vi "Com_Test.vi"() -> ()   [LabVIEW 2020]
uses:
  <vilib>/Instr/_visa.llb/VISA Configure Serial Port (Serial Instr).vi
panel:
  out "missed msg":u16
  out "error out":errorcluster
  out "error cleared?":bool
  out "Next Cmd":enum16{"getParm", "inc", "mph", "err"}(ring)
  out "Next State":enum16{"Initialize", "Send", "Receive", "Error"}(ring)
  out "stopping":bool
  out "Target MPH":u16 max=12 step=1 format="%2d"
  out "step":i32
  out "Target INC":u16 max=12 step=1
  out "Speed Changed":bool
  out "Inc Changed":bool
  in  "stop":bool
  out "read buffer":string
  out "refnum out":refnum<file>
  out "MPH READ":u8
  out "MPH READ 2":u8
  out "INC READ":u8
  out "INC READ 2":u8
  out "PD READ":u8 format="%x"
  out "PD READ 2":u8 format="%x"
  in  "Serial Port":refnum<visa-resource-name>="COM8"
  out "FootPath":path
  out "FootPathRef":refnum<file>
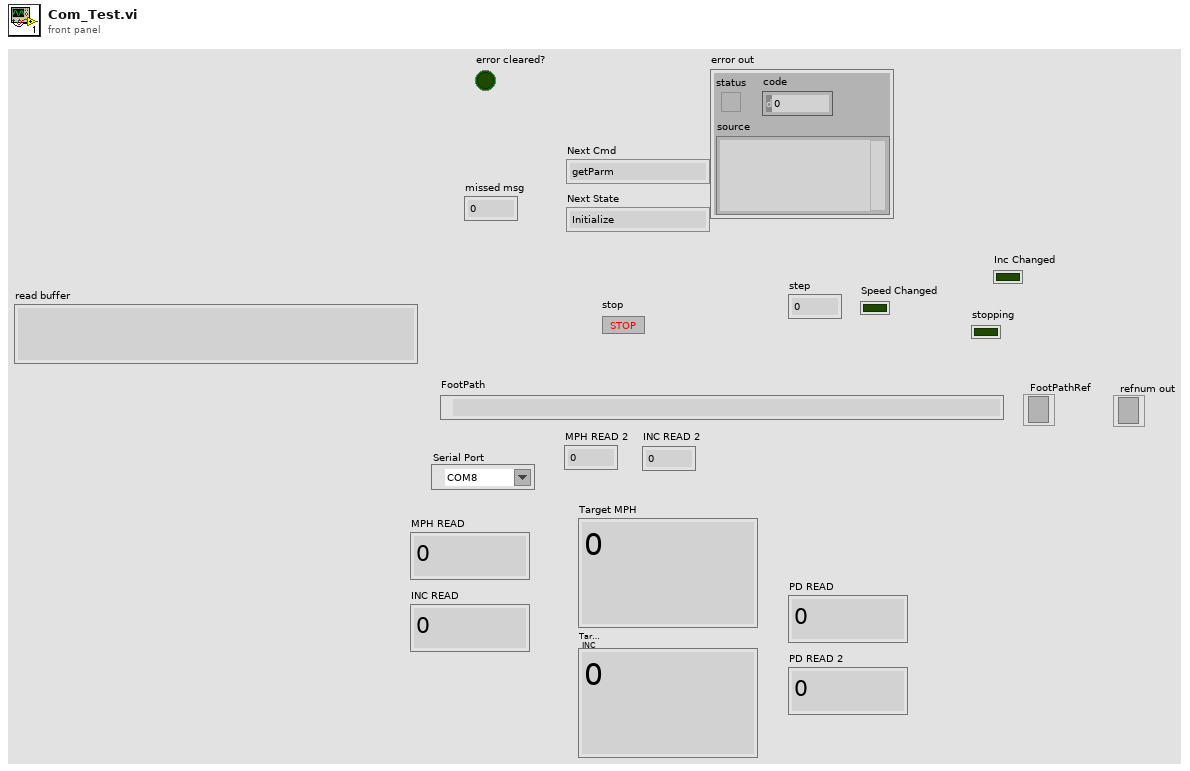
[diagram p1: front panel]
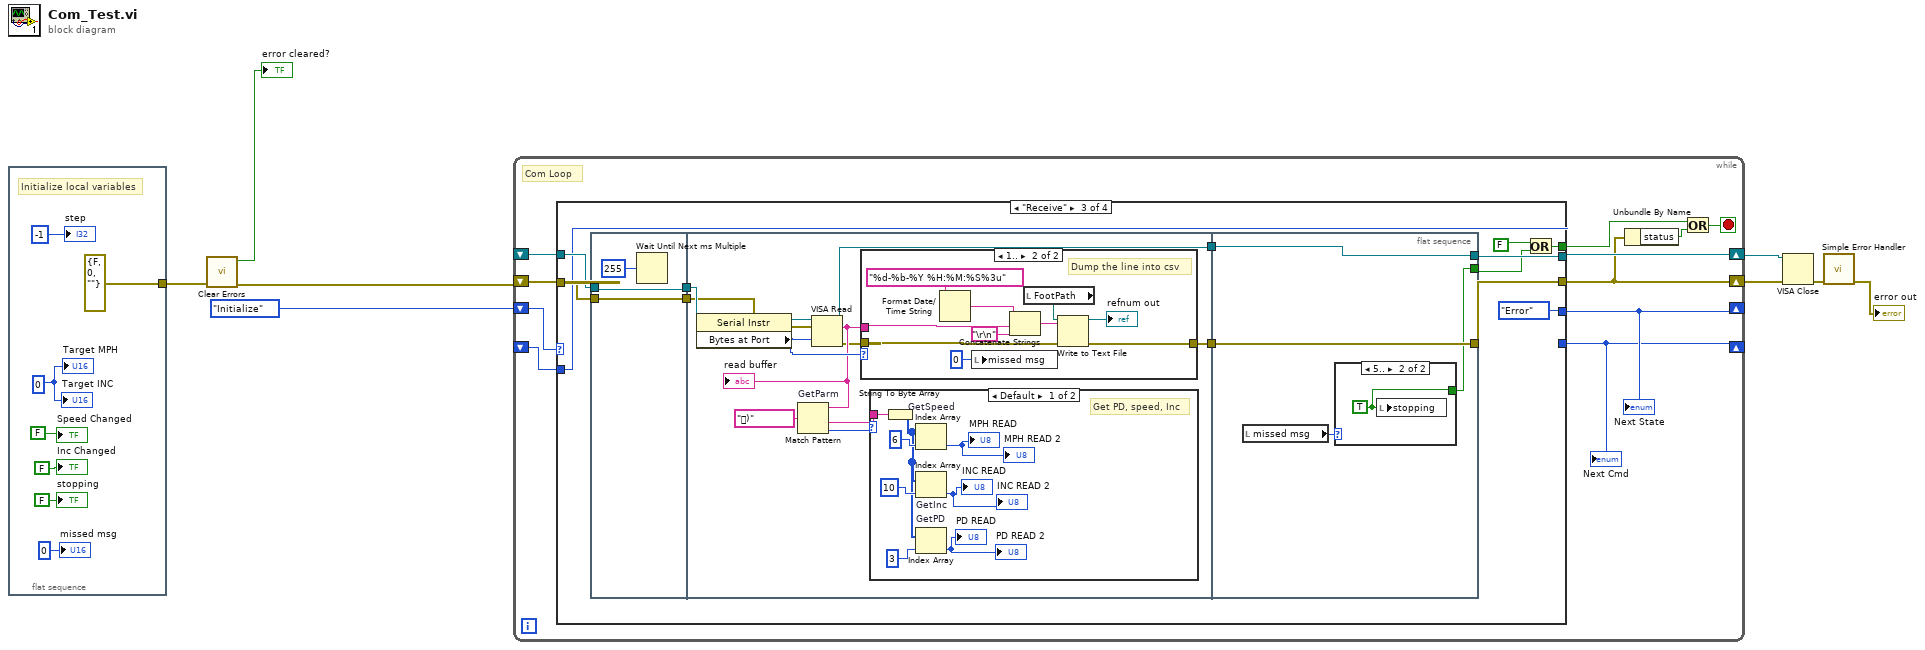
[diagram p0: block diagram]
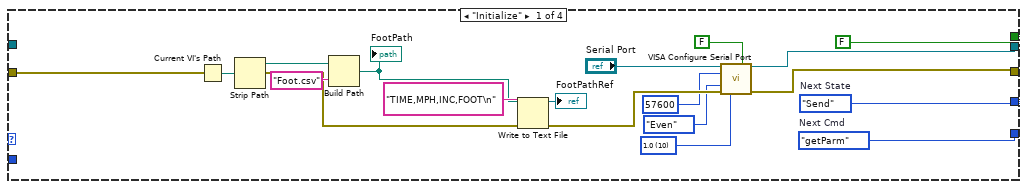
[diagram p2: hidden frame]
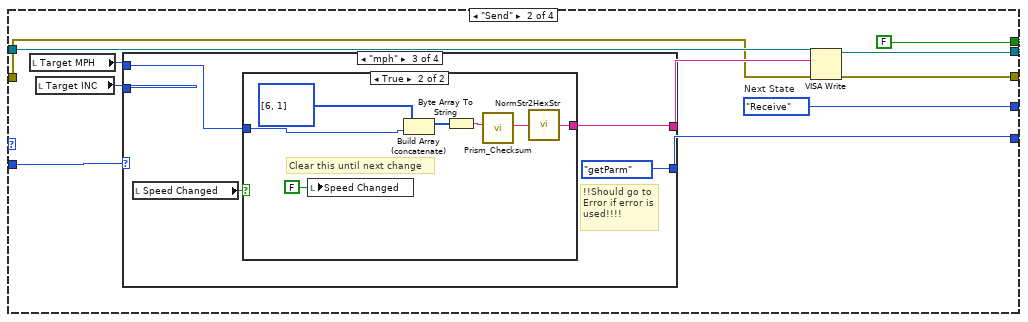
[diagram p3: hidden frame]
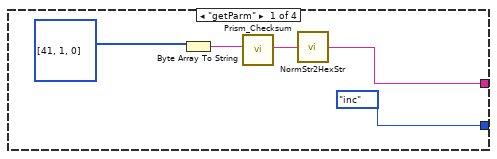
[diagram p4: hidden frame]
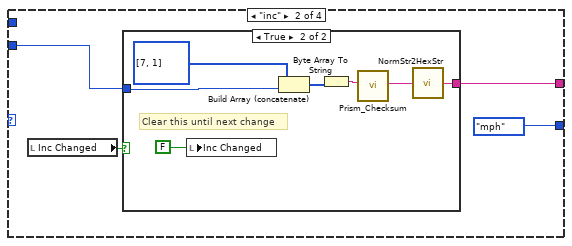
[diagram p5: hidden frame]
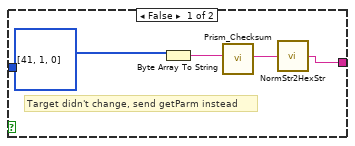
[diagram p6: hidden frame]
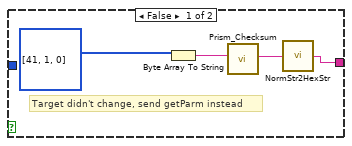
[diagram p7: hidden frame]
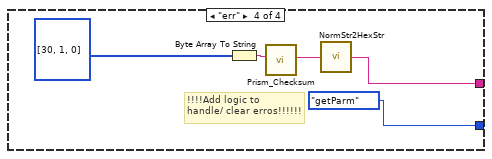
[diagram p8: hidden frame]
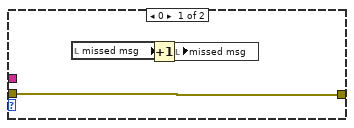
[diagram p10: hidden frame]
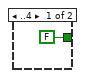
[diagram p11: hidden frame]
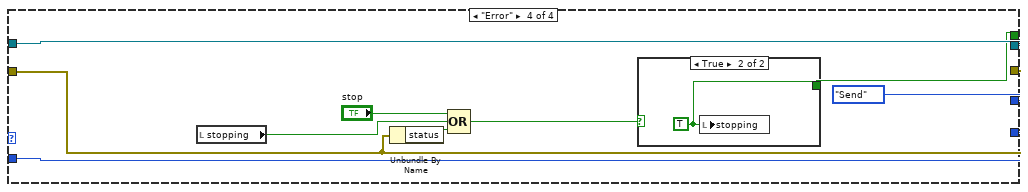
[diagram p12: hidden frame]
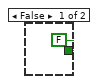
[diagram p13: hidden frame]
diagram:
  n1 = flat-sequence {
    tunnel: [errorcluster {"status"=FALSE, "code"=0, "source"=""} ("error constant")] -> w4
    frame #0 {
      w11 = u16 0 ("MPH")
      # "Initialize local variables"
      "stopping" <- FALSE ("stopping")
      "Target MPH" <- w11
      "step" <- -1 ("step")
      "Target INC" <- w11
      "Speed Changed" <- FALSE ("Value Changed")
      "Inc Changed" <- FALSE ("Inc Changed")
      "missed msg" <- u16 0 ("0 bytes")
    }
  }
  n2 = call <vilib>:"Clear Errors.vi"("error in (no error)"=w4) -> ("error out"=w3:errorcluster, "specific error cleared?"=→"error cleared?":bool)  [unwired: 5 in]
  n3 = while {
    shift-right: [w18] -> w7
    shift-left: w3 -> [w26]
    shift-right: [w23] -> w6
    shift-left: _ -> [w25]
    shift-right: [w22] -> _
    shift-left: enum16{"Initialize", "Send", "Receive", "Error"}."Initialize" ("Next State") -> [w24]
    shift-right: [w21] -> _
    shift-left: _ -> [w20]
    stop <- w17 stop-if-true
    # "Com Loop"
    n4 = case shown="\"Receive\"" w24 {
      tunnel: w26 -> [w32 w46 w106 w152]
      tunnel: w25 -> [_ w53 w108 w157]
      tunnel: [w42 w55 w101 w157] -> w23
      tunnel: [w41 w54 w102 w152] -> w18
      tunnel: [w38 w49 enum16{"Initialize", "Send", "Receive", "Error"}."Error" enum16{"Initialize", "Send", "Receive", "Error"}."Send"] -> w22
      tunnel: [w40 w47 w105 w158] -> w21
      tunnel: w20 -> [_ w45 w105 w158]
      tunnel: [FALSE FALSE w98 w153] -> w19
      frame "Initialize" {
        w27 = u16 10 items=["1.0"=10, "1.5"=15, "2.0"=20] ("stop bits (10: 1 bit)")
        w38 = enum16{"Initialize", "Send", "Receive", "Error"}."Send"  # Next State
        w40 = enum16{"getParm", "inc", "mph", "err"}."getParm"  # Next Cmd
        n5 = Current VI's Path() -> (path=w37:path)
        n6 = Strip Path(path=w37) -> (stripped path=w36:path)  [unwired: 1 out]
        n7 = Build Path(base path=w36, name or relative path="Foot.csv") -> (appended path=w33:path)
        "FootPath" <- w33
        n8 = Write to Text File(file (use dialog)=w33, text="TIME,MPH,INC,FOOT\n", error in=w32) -> (refnum out=→"FootPathRef":refnum<file>, error out=w31:errorcluster)  [unwired: 1 in, 1 out]
        n9 = call-poly "VISA Configure Serial Port"("VISA resource name"="Serial Port", "Enable Termination\nChar (T)"=FALSE ("Enable Termination\nChar (T)"), "baud rate (9600)"=u32 57600, "parity (0:none)"=enum16{"None", "Odd", "Even", "Mark", "Space"}."Even", "error in (no error)"=w31, "stop bits (10: 1 bit)"=w27) -> ("VISA resource name out"=w42:refnum<visa-resource-name>, "error out"=w41:errorcluster)  [unwired: 8 in]
      }
      frame "Send" {
        w49 = enum16{"Initialize", "Send", "Receive", "Error"}."Receive"  # Next State
        n10 = local read "Target MPH"() -> (w51:u16)
        n11 = local read "Target INC"() -> (w50:u16)
        n12 = case shown="\"mph\"" w45 {
          tunnel: w51 -> [_ _ w77 _]
          tunnel: w50 -> [_ w64 _ _]
          tunnel: [w56 w63 w78 w92] -> w48
          tunnel: [enum16{"getParm", "inc", "mph", "err"}."inc" enum16{"getParm", "inc", "mph", "err"}."mph" enum16{"getParm", "inc", "mph", "err"}."getParm" enum16{"getParm", "inc", "mph", "err"}."getParm"] -> w47
          frame "getParm" {
            n13 = Byte Array To String(unsigned byte array=u8[] [41, 1, 0]) -> (string=w58:string)
            n14 = call "Prism_Checksum.vi"("ID +DB+ Data"=w58) -> ("Full Cmd"=w57:string)  [unwired: 10 in]
            n15 = call "NormStr2HexStr.vi"("string"=w57) -> ("hex string"=w56:string)
          }
          frame "inc" {
            n16 = local read "Inc Changed"() -> (w61:bool)
            n17 = case shown="True" w61 {
              tunnel: w64 -> [_ w72]
              tunnel: [w65 w70] -> w63
              frame False {
                # "Target didn't change, send getParm instead"
                n18 = Byte Array To String(unsigned byte array=u8[] [41, 1, 0]) -> (string=w67:string)
                n19 = call "Prism_Checksum.vi"("ID +DB+ Data"=w67) -> ("Full Cmd"=w66:string)  [unwired: 10 in]
                n20 = call "NormStr2HexStr.vi"("string"=w66) -> ("hex string"=w65:string)
              }
              frame True {
                # "Clear this until next change"
                n21 = local write "Inc Changed"(FALSE ("Value Changed")) -> ()
                n22 = Build Array (concatenate)(u8[] [7, 1] ("unsigned byte array"), w72) -> (w71:u16[])
                n23 = Byte Array To String(unsigned byte array=w71) -> (string=w74:string)
                n24 = call "Prism_Checksum.vi"("ID +DB+ Data"=w74) -> ("Full Cmd"=w75:string)  [unwired: 10 in]
                n25 = call "NormStr2HexStr.vi"("string"=w75) -> ("hex string"=w70:string)
              }
            }
          }
          frame "mph" {
            # "!!Should go to\nError if error is\nused!!!!"
            n26 = local read "Speed Changed"() -> (w76:bool)
            n27 = case shown="True" w76 {
              tunnel: [w80 w87] -> w78
              tunnel: w77 -> [_ w85]
              frame False {
                # "Target didn't change, send getParm instead"
                n28 = Byte Array To String(unsigned byte array=u8[] [41, 1, 0]) -> (string=w82:string)
                n29 = call "Prism_Checksum.vi"("ID +DB+ Data"=w82) -> ("Full Cmd"=w81:string)  [unwired: 10 in]
                n30 = call "NormStr2HexStr.vi"("string"=w81) -> ("hex string"=w80:string)
              }
              frame True {
                # "Clear this until next change"
                n31 = local write "Speed Changed"(FALSE ("Value Changed")) -> ()
                n32 = Build Array (concatenate)(u8[] [6, 1] ("unsigned byte array"), w85) -> (w86:u16[])
                n33 = Byte Array To String(unsigned byte array=w86) -> (string=w89:string)
                n34 = call "Prism_Checksum.vi"("ID +DB+ Data"=w89) -> ("Full Cmd"=w90:string)  [unwired: 10 in]
                n35 = call "NormStr2HexStr.vi"("string"=w90) -> ("hex string"=w87:string)
              }
            }
          }
          frame "err" {
            # "!!!!Add logic to\nhandle/ clear erros!!!!!!"
            n36 = Byte Array To String(unsigned byte array=u8[] [30, 1, 0]) -> (string=w94:string)
            n37 = call "Prism_Checksum.vi"("ID +DB+ Data"=w94) -> ("Full Cmd"=w95:string)  [unwired: 10 in]
            n38 = call "NormStr2HexStr.vi"("string"=w95) -> ("hex string"=w92:string)
          }
        }
        n39 = VISA Write(VISA resource name=w53, write buffer=w48, error in (no error)=w46) -> (VISA resource name out=w55:refnum<visa-resource-name>, error out=w54:errorcluster)  [unwired: 1 out]
      }
      frame "Receive" {
        n40 = flat-sequence {
          tunnel: w108 -> [w110]
          tunnel: w106 -> [w109]
          tunnel: [w110] -> w104
          tunnel: [w109] -> w103
          tunnel: w104 -> [w115]
          tunnel: w103 -> [w114]
          tunnel: [w113] -> w100
          tunnel: [w112] -> w99
          tunnel: [w147] -> w101
          tunnel: [w148] -> w102
          tunnel: w100 -> [w148]
          tunnel: w99 -> [w147]
          tunnel: [w145] -> w96
          frame #0 {
            n41 = Wait Until Next ms Multiple(millisecond multiple=u32 255) -> ()  [unwired: 1 out]
          }
          frame #1 {
            n42 = property class="Serial Instr"(reference=w115, error in=w114) -> (reference out=w118:refnum<visa-resource-name>, error out=w117:errorcluster, "Bytes at Port"=w123:u32)
            n43 = VISA Read(VISA resource name=w118, byte count=w123, error in (no error)=w117) -> (VISA resource name out=w112:refnum<visa-resource-name>, read buffer=w122:string, error out=w119:errorcluster)  [unwired: 1 out]
            "read buffer" <- w122
            n44 = Match Pattern "GetParm"(string=w122, regular expression="ޭ)") -> (after substring=w121:string, offset past match=w120:i32)  [unwired: 1 in, 2 out]
            n45 = case shown="1.." w123 {
              tunnel: w122 -> [_ w138]
              tunnel: [w134 w137] -> w113
              tunnel: w119 -> [w134 w136]
              frame 0 {
                n46 = local read "missed msg"() -> (w133:u16)
                n47 = Increment(x=w133) -> (x+1=w132:u16)
                n48 = local write "missed msg"(w132) -> ()
              }
              frame 1.. {
                # "Dump the line into csv"
                n49 = Format Date/Time String(time format string (%c)="%d-%b-%Y %H:%M:%S%3u") -> (date/time string=w144:string)  [unwired: 2 in]
                n50 = local write "missed msg"(u16 0 ("missed msg")) -> ()
                n51 = Concatenate Strings(w144, w138, "\r\n") -> (w141:string)
                n52 = local read "FootPath"() -> (w142:path)
                n53 = Write to Text File(file (use dialog)=w142, text=w141, error in=w136) -> (refnum out=→"refnum out":refnum<file>, error out=w137:errorcluster)  [unwired: 1 in, 1 out]
              }
            }
            n54 = case shown="Default" w120 {
              tunnel: w121 -> [w131 _]
              frame Default {
                # "Get PD, speed, Inc"
                n55 = String To Byte Array(string=w131) -> (unsigned byte array=w125:u8[])
                n56 = Index Array "GetSpeed"(array=w125, index=6) -> (element=→"MPH READ" →"MPH READ 2":u8)
                n57 = Index Array "GetInc"(array=w125, index=10) -> (element=→"INC READ" →"INC READ 2":u8)
                n58 = Index Array "GetPD"(array=w125, index=3) -> (element=→"PD READ" →"PD READ 2":u8)
              }
              frame -1 {
              }
            }
          }
          frame #2 {
            n59 = local read "missed msg"() -> (w146:u16)
            n60 = case shown="5.." w146 {
              tunnel: [FALSE ("stopping") w150] -> w145
              frame ..4 {
              }
              frame 5.. {
                w150 = TRUE ("stopping")
                n61 = local write "stopping"(w150) -> ()
              }
            }
          }
        }
        n62 = Or(x=FALSE, y=w96) -> (x .or. y?=w98:bool)
      }
      frame "Error" {
        n63 = local read "stopping"() -> (w154:bool)
        n64 = Unbundle By Name(w152) -> ("status"=w151:bool)
        n65 = Compound Arithmetic op=OR("stop", w154, w151) -> (w156:bool)
        n66 = case shown="True" w156 {
          tunnel: [FALSE w161] -> w153
          frame False {
          }
          frame True {
            w161 = TRUE ("stopping")
            n67 = local write "stopping"(w161) -> ()
          }
        }
      }
    }
    "Next State" <- w22
    "Next Cmd" <- w21
    n68 = Unbundle By Name(w18) -> ("status"=w16:bool)
    n69 = Or(x=w19, y=w16) -> (x .or. y?=w17:bool)
  }
  n70 = VISA Close(VISA resource name=w6, error in (no error)=w7) -> (error out=w8:errorcluster)
  n71 = call <vilib>:"Simple Error Handler.vi"("error in (no error)"=w8) -> ("error out"=→"error out":errorcluster)  [unwired: 4 in, 4 out]
